vi "UI.vi"() -> ()   [LabVIEW 2015]
uses:
  Facade/cPAS Facade.lvclass
  Facade/Data.ctl
  Reusable/Commands/Command.lvclass
  Devices/Alicat/Session Based/Data/M/M data.lvclass
  Devices/Alicat/Session Based/Data/MC/MC Data.lvclass
  Reusable/GUI/Facade/GUI Facade.lvclass/GUI Facade.ctl
  Controls/Flags.ctl
  Reusable/Data/Read measTime.vi
  Reusable/GUI/Facade/GUI Facade.lvclass
  Reusable/Data/Data.lvclass
  Reusable/Error Logging/Error Logger.lvclass
panel:
  in  "swDispl":T1={"mDispl"=TRUE, "crdCtl"=FALSE, "pasCtl"=FALSE, "housekeeping"=FALSE, "crdRD"=FALSE, "pasSig"=FALSE, "power"=FALSE, "power 2"=FALSE, "power 3"=FALSE, "power 4"=FALSE}
  in  "saveRDs":bool
  out "Version":string
  in  "Sync Time":bool
  out "filter?":bool caption="Filter?"
  out "PAS Time Good":bool
  out "CRD Time Good":bool
  out "filtTime":timestamp caption="Last Filter Switch" format="%<%H:%M:%S>T"
  out "pasTime":timestamp caption="PAS Time" format="%<%H:%M:%S>T"
  out "crdTime":timestamp caption="CRD Time" format="%<%H:%M:%S>T"
  in  "filter":bool
  out "General Error":bool
  out "CRD Error":bool
  out "PAS Error":bool
  out "Saving":bool
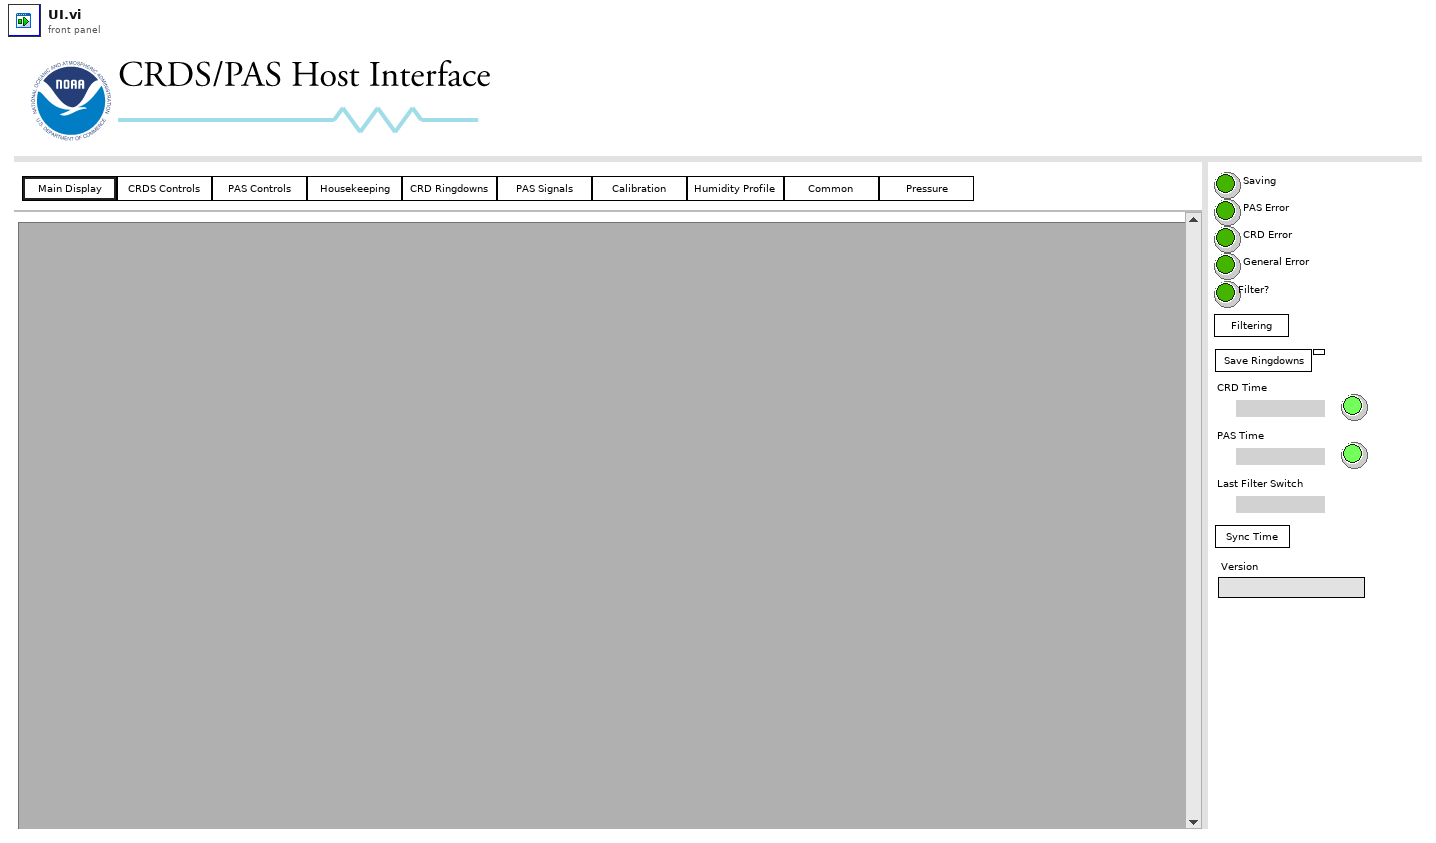
[diagram p1: front panel]
types:
  T1 = cluster{"mDispl":bool, "crdCtl":bool, "pasCtl":bool, "housekeeping":bool, "crdRD":bool, "pasSig":bool, "power":bool, "power 2":bool, "power 3":bool, "power 4":bool}
  T2 = enum8{"Enabled", "Disabled", "Disabled and Grayed Out"}
  T3 = typedef "cPAS Facade.lvclass/Data.ctl" = enum16{"PAS", "CRD", "CLAP"}
  T4 = typedef "Flags.ctl" = enum8{"Autospeaker", "Link cycles", "Autofilter", "O3 Cal", "Filter Position"}
  T5 = cluster{"[0]":bool, "[1]":bool, "[2]":bool, "[3]":bool, "[4]":bool, "[5]":bool, "[6]":bool, "[7]":bool, "[8]":bool, "[9]":bool}
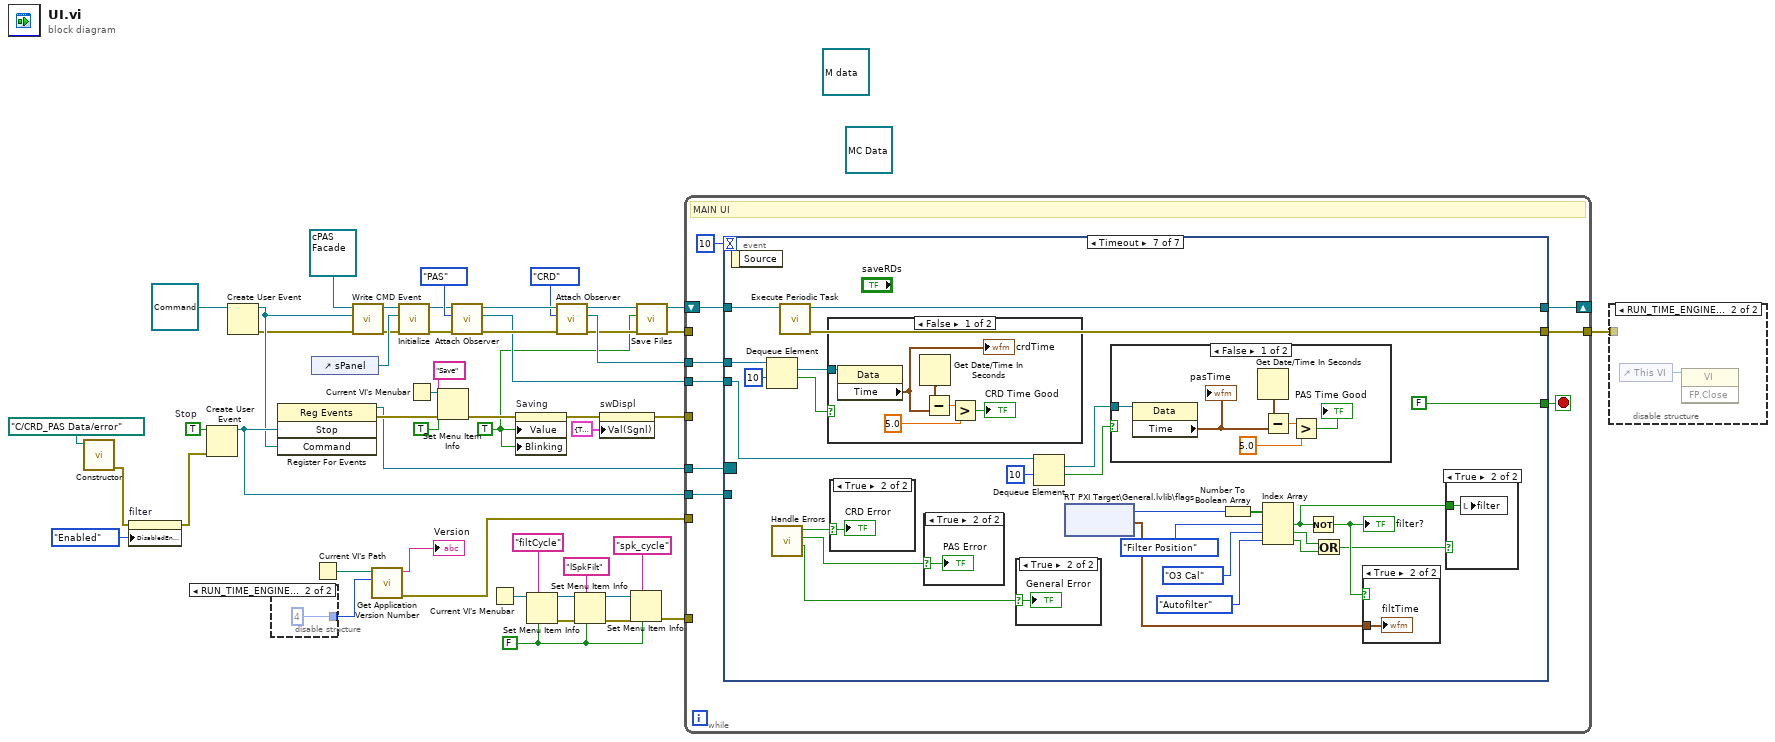
[diagram p0: block diagram]
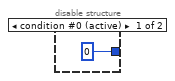
[diagram p2: hidden frame]
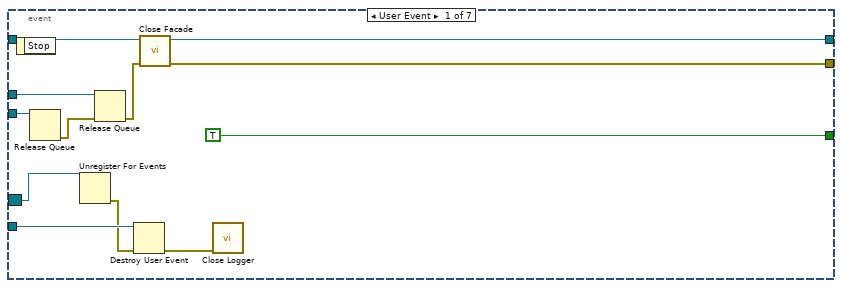
[diagram p4: hidden frame]
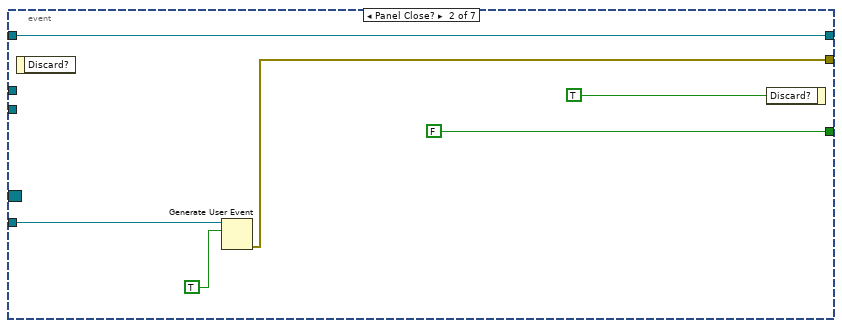
[diagram p5: hidden frame]
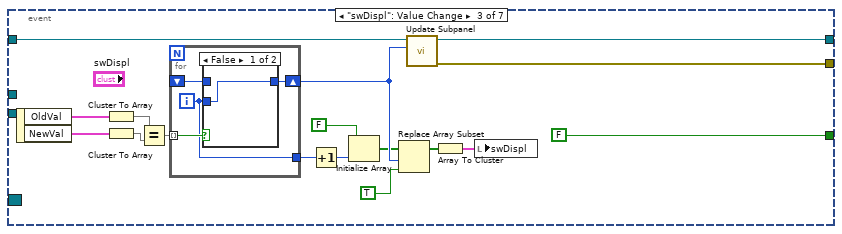
[diagram p6: hidden frame]
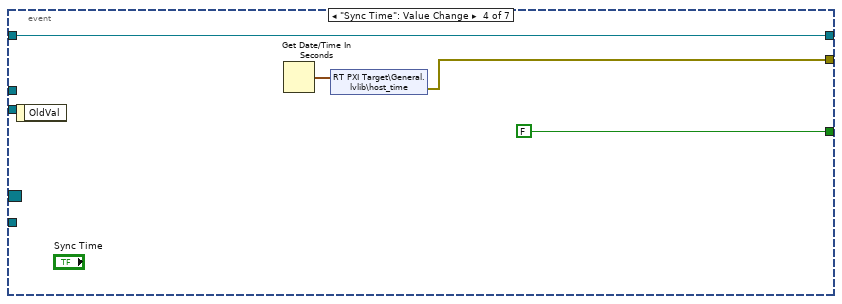
[diagram p8: hidden frame]
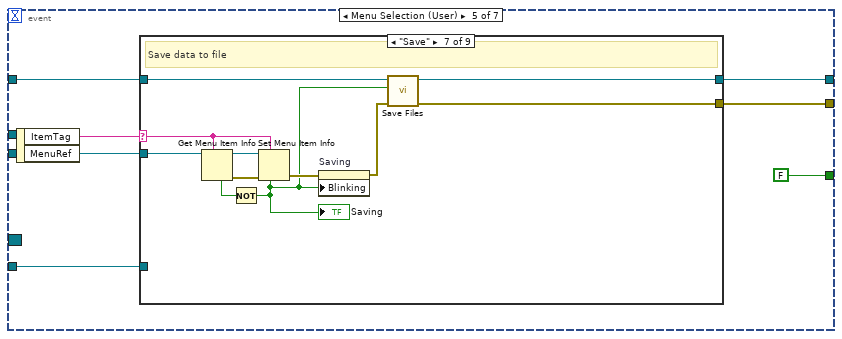
[diagram p9: hidden frame]
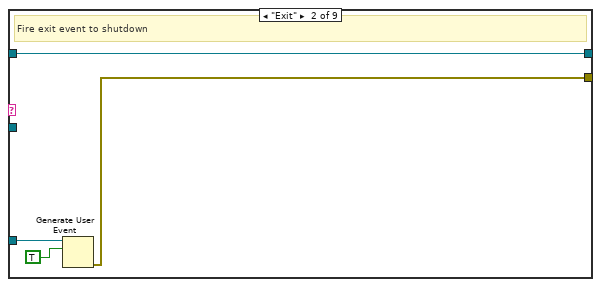
[diagram p11: hidden frame]
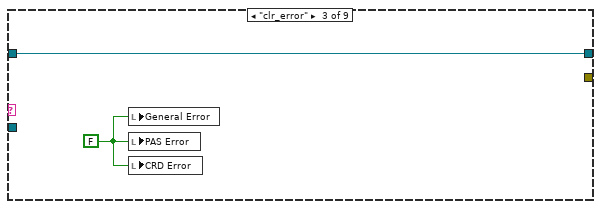
[diagram p12: hidden frame]
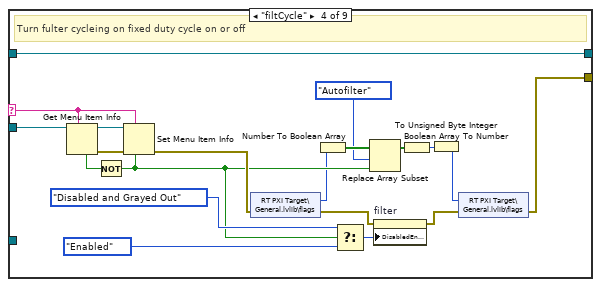
[diagram p13: hidden frame]
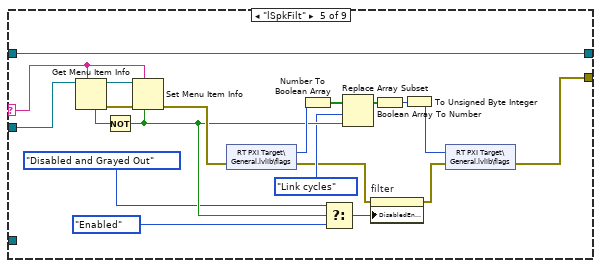
[diagram p14: hidden frame]
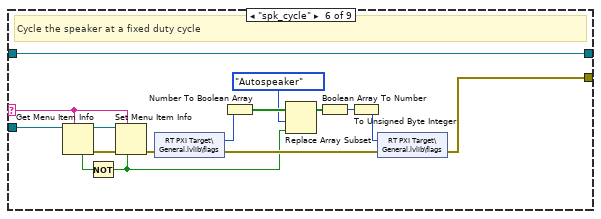
[diagram p15: hidden frame]
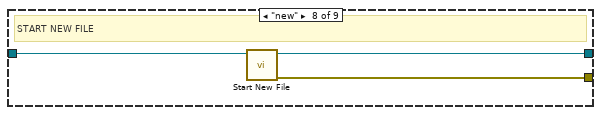
[diagram p16: hidden frame]
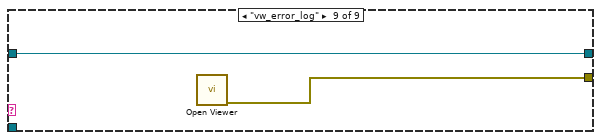
[diagram p17: hidden frame]
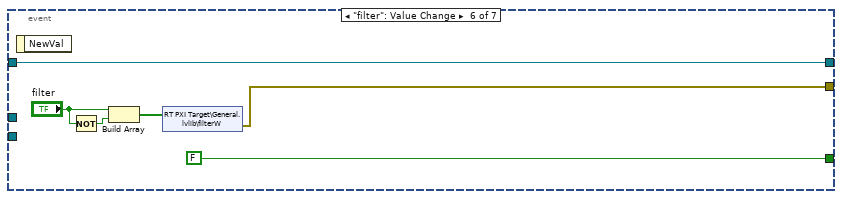
[diagram p18: hidden frame]
diagram:
  (unwired) refnum<class "MC Data.lvclass"> refnum ("MC Data")
  (unwired) refnum<class "M data.lvclass"> refnum ("M Data")
  w8 = FALSE ("checked")
  w39 = TRUE  # Stop
  w32 = TRUE ("Saving")
  n1 = call "Constructor.vi"("Main Path"=path "C:/CRD_PAS Data/error" ("Data Path")) -> ("error out"=w6:errorcluster)  [unwired: 10 in]
  n2 = property on="filter" class="Bool (strict)"(error in=w6, "DisabledEnum"=T2."Enabled" ("Disabled")) -> (error out=w17:errorcluster)  [unwired: 1 in, 1 out]
  n3 = Create User Event(user event datatype=w39, error in=w17) -> (user event=w37:refnum<user-event>)  [unwired: 1 out]
  n4 = Create User Event(user event datatype=refnum<class "Command.lvclass"> refnum ("Command")) -> (user event=w21:refnum<user-event>, error out=w19:errorcluster)  [unwired: 1 in]
  n5 = disable-structure shown="RUN_TIME_ENGINE==True" {
    disable-tunnel: [0 ("Number to Strip") 4 ("Number to Strip")] -> w4
    frame condition #0 (active) {
    }
    frame condition #1 {
    }
  }
  n6 = register-events(w37, w21) -> (reference out=w27:refnum<event-registration>, error out=w38:errorcluster)  [unwired: 2 in]
  n7 = control-ref of="sPanel"() -> (w46:refnum<vi>)
  n8 = Current VI's Path() -> (path=w5:path)
  n9 = call "Write CMD Event.vi"("error in (no error)"=w19, "CMD Event"=w21, "GUI Facade in"=refnum<class "cPAS Facade.lvclass"> refnum ("cPAS Facade")) -> ("error out"=w22:errorcluster, "GUI Facade out"=w23:refnum<class "cPAS Facade.lvclass">)  [unwired: 7 in]
  n10 = call "Get Application Version Number.vi"("Number to Strip"=w4, "Initial Path"=w5) -> ("error out"=w3:errorcluster, "Version"=→"Version":string)  [unwired: 8 in]
  n11 = call-dynamic "Initialize.vi"("error in"=w22, "sPanel"=w46, "GUI Facade in"=w23) -> ("error out"=w1:errorcluster, "GUI Facade out"=w20:refnum<class "cPAS Facade.lvclass">)  [unwired: 7 in]
  n12 = Current VI's Menubar() -> (w50:refnum<k9>)
  n13 = Set Menu Item Info(6:TRUE ("checked"), 7:"Save" ("item tag"), 8:w38, 11:w50) -> (0:w47:errorcluster)  [unwired: 3 in, 1 out]
  n14 = call "Attach Observer.vi"("error in"=w1, "Subject"=Data."PAS" ("Data"), "GUI Facade in"=w20) -> ("error out"=w44:errorcluster, "Observer"=w40:refnum<queue>, "GUI Facade out"=w45:refnum<class "cPAS Facade.lvclass">)  [unwired: 6 in]
  n15 = Current VI's Menubar() -> (w16:refnum<k9>)
  n16 = property on="Saving" class="Bool (strict)"(error in=w47, "Value"=w32, "Blinking"=w32) -> (error out=w30:errorcluster)  [unwired: 1 in, 1 out]
  n17 = Set Menu Item Info(6:w8, 7:"filtCycle" ("item tag"), 11:w16) -> (0:w12:errorcluster, 3:w13:refnum<k9>)  [unwired: 4 in]
  n18 = call "Attach Observer.vi"("error in"=w44, "Subject"=Data."CRD" ("Data"), "GUI Facade in"=w45) -> ("error out"=w34:errorcluster, "Observer"=w41:refnum<queue>, "GUI Facade out"=w36:refnum<class "cPAS Facade.lvclass">)  [unwired: 6 in]
  n19 = Set Menu Item Info(6:w8, 7:"lSpkFilt" ("item tag"), 8:w12, 11:w13) -> (0:w10:errorcluster, 3:w11:refnum<k9>)  [unwired: 3 in]
  n20 = property on="swDispl" class="Clust (strict)"(error in=w30, "Val(Sgnl)"=T1 {"mDispl"=TRUE, "crdCtl"=FALSE, "pasCtl"=FALSE, "housekeeping"=FALSE, "crdRD"=FALSE, "pasSig"=FALSE, "power"=FALSE, "power 2"=FALSE, "power 3"=FALSE, "power 4"=FALSE} ("Value (Signaling)")) -> (error out=w29:errorcluster)  [unwired: 1 in, 1 out]
  n21 = Set Menu Item Info(6:w8, 7:"spk_cycle" ("item tag"), 8:w10, 11:w11) -> (0:w7:errorcluster)  [unwired: 3 in, 1 out]
  n22 = call "Save Files.vi"("error in"=w34, "Write"=w32, "GUI Facade in"=w36) -> ("error out"=w33:errorcluster, "GUI Facade out"=w35:refnum<class "cPAS Facade.lvclass">)  [unwired: 7 in]
  n23 = while {
    shift-right: [w58] -> _
    shift-left: w35 -> [w59]
    tunnel: w41 -> [w57]
    tunnel: w40 -> [w56]
    tunnel: w27 -> [w55]
    tunnel: w37 -> [w54]
    tunnel: [w53] -> w28
    tunnel: w33 -> [_]
    tunnel: w29 -> [_]
    tunnel: w7 -> [_]
    tunnel: w3 -> [_]
    stop <- w61 stop-if-true
    # "MAIN UI"
    n24 = event shown="[6] Timeout" {
      selector: w55 -> [w65 _ _ _ _ _ _]
      dyn-events: _ -> [_ _ _ _ _ _ _]
      timeout: 10 -> [_ _ _ _ _ _ _]
      tunnel: [TRUE ("stop") FALSE ("stop") FALSE ("stop") FALSE ("stop") FALSE ("stop") FALSE ("stop") FALSE ("stop")] -> w61
      tunnel: [w71 w76 w92 w103 w111 w197 w223] -> w53
      tunnel: w59 -> [w72 w75 w93 w106 w110 w196 w224]
      tunnel: [w70 w75 w91 w106 w109 w196 w222] -> w58
      tunnel: w57 -> [w68 _ _ _ _ _ w218]
      tunnel: w56 -> [w69 _ _ _ _ _ w216]
      tunnel: w54 -> [w64 w77 _ _ w108 _ _]
      event User Event {
        n25 = event-data() -> ()  [unwired: 1 in, 1 out]
        n26 = Release Queue(queue=w69) -> (error out=w67:errorcluster)  [unwired: 2 in, 2 out]
        n27 = Unregister For Events(event registration refnum=w65) -> (error out=w63:errorcluster)  [unwired: 1 in]
        n28 = Release Queue(queue=w68, error in (no error)=w67) -> (error out=w66:errorcluster)  [unwired: 1 in, 2 out]
        n29 = Destroy User Event(user event=w64, error in=w63) -> (error out=w62:errorcluster)
        n30 = call-dynamic "Close Facade.vi"("error in"=w66, "cPAS Facade in"=w72) -> ("error out"=w71:errorcluster, "cPAS Facade out"=w70:refnum<class "cPAS Facade.lvclass">)  [unwired: 8 in]
        n31 = call "Close Logger.vi"("error in"=w62) -> ()  [unwired: 9 in, 2 out]
      }
      event Panel Close? {
        n32 = event-data() -> ()  [unwired: 1 in, 1 out]
        n33 = Generate User Event(user event=w77, event data cluster=TRUE ("event data")) -> (error out=w76:errorcluster)  [unwired: 2 in, 1 out]
        n34 = event-data("Discard?"=TRUE) -> ()  [unwired: 1 in, 1 out]
      }
      event "swDispl": Value Change {
        n35 = event-data() -> ("OldVal"=w96:T1, "NewVal"=w95:T1)  [unwired: 1 in]
        n36 = Cluster To Array(cluster=w96) -> (array=w89:bool[])
        n37 = Cluster To Array(cluster=w95) -> (array=w90:bool[])
        n38 = Equal?(x=w89, y=w90) -> (x = y?=w94:bool[])
        n39 = for {
          tunnel: w94 -> [w100] mode=indexing
          shift-right: [w99] -> w85
          shift-left: _ -> [w98]
          tunnel: [w97] -> w88
          i -> [w97]
          n40 = case shown="False" w100 {
            tunnel: w97 -> [w101 _]
            tunnel: [w101 w102] -> w99
            tunnel: w98 -> [_ w102]
            frame False {
            }
            frame True {
            }
          }
        }
        n41 = Increment(x=w88) -> (x+1=w87:i32)
        n42 = Initialize Array(FALSE, w87) -> (w84:bool[])
        n43 = Replace Array Subset(array=w84, new element=TRUE ("new element/subarray"), index=w85) -> (w82:bool[])
        n44 = call "Update Subpanel.vi"("sPanel"=w85, "GUI Facade in"=w93) -> ("error out"=w92:errorcluster, "GUI Facade out"=w91:refnum<class "cPAS Facade.lvclass">)  [unwired: 8 in]
        n45 = Array To Cluster(array=w82) -> (cluster=w81:T5)
        n46 = local write "swDispl"(w81) -> ()
      }
      event "Sync Time": Value Change {
        n47 = event-data() -> ()  [unwired: 1 in, 1 out]
        n48 = Get Date/Time In Seconds() -> (seconds since 1Jan1904=w104:timestamp)
        n49 = shared-variable "RT PXI Target\\General.lvlib\\host_time"(w104) -> (error out=w103:errorcluster)  [unwired: 1 in]
      }
      event Menu Selection (User) {
        n50 = event-data() -> ("ItemTag"=w112:string, "MenuRef"=w113:refnum<k9>)  [unwired: 1 in]
        n51 = case shown="\"Save\"" w112 {
          selector: w112 -> [_ _ _ w136 w147 w165 w182 _ _]
          tunnel: w113 -> [_ _ _ w135 w146 w166 w183 _ _]
          tunnel: [_ w115 _ w133 w144 w164 w177 w188 w191] -> w111
          tunnel: [w114 w118 w119 w140 w145 w163 w180 w189 w192] -> w109
          tunnel: w110 -> [w114 w118 w119 w140 w145 w163 w181 w190 w192]
          tunnel: w108 -> [_ w117 _ _ _ _ _ _ _]
          frame "NULL", Default {
            # "Do Nothing"
          }
          frame "Exit" {
            # "Fire exit event to shutdown"
            n52 = Generate User Event(user event=w117, event data cluster=TRUE ("event data")) -> (error out=w115:errorcluster)  [unwired: 2 in, 1 out]
          }
          frame "clr_error" {
            w120 = FALSE
            n53 = local write "General Error"(w120) -> ()
            n54 = local write "PAS Error"(w120) -> ()
            n55 = local write "CRD Error"(w120) -> ()
          }
          frame "filtCycle" {
            # "Turn fulter cycleing on fixed duty cycle on or off"
            n56 = Get Menu Item Info(7:w136, 11:w135) -> (0:w137:errorcluster, 3:w138:refnum<k9>, 4:w139:bool)  [unwired: 1 in, 4 out]
            n57 = Not(x=w139) -> (.not. x?=w129:bool)
            n58 = Set Menu Item Info(6:w129, 7:w136, 8:w137, 11:w138) -> (0:w134:errorcluster)  [unwired: 3 in, 1 out]
            n59 = shared-variable "RT PXI Target\\General.lvlib\\flags"(error in=w134) -> (w124:u8, error out=w122:errorcluster)
            n60 = Number To Boolean Array(number=w124) -> (Boolean array=w125:bool[])
            n61 = Select(t=T2."Disabled and Grayed Out", s=w129, f=T2."Enabled" ("Disabled")) -> (s? t:f=w130:T2)
            n62 = Replace Array Subset(array=w125, new element=w129, index=Flags."Autofilter" ("Flags")) -> (w126:bool[])
            n63 = property on="filter" class="Bool (strict)"(error in=w122, "DisabledEnum"=w130) -> (error out=w121:errorcluster)  [unwired: 1 in, 1 out]
            n64 = Boolean Array To Number(Boolean array=w126) -> (number=w127:u32)
            n65 = To Unsigned Byte Integer(number=w127) -> (unsigned 8bit integer=w128:u8)
            n66 = shared-variable "RT PXI Target\\General.lvlib\\flags"(w128, error in=w121) -> (error out=w133:errorcluster)
          }
          frame "lSpkFilt" {
            n67 = Get Menu Item Info(7:w147, 11:w146) -> (0:w158:errorcluster, 3:w159:refnum<k9>, 4:w160:bool)  [unwired: 1 in, 4 out]
            n68 = Not(x=w160) -> (.not. x?=w150:bool)
            n69 = Set Menu Item Info(6:w150, 7:w147, 8:w158, 11:w159) -> (0:w152:errorcluster)  [unwired: 3 in, 1 out]
            n70 = shared-variable "RT PXI Target\\General.lvlib\\flags"(error in=w152) -> (w153:u8, error out=w142:errorcluster)
            n71 = Number To Boolean Array(number=w153) -> (Boolean array=w154:bool[])
            n72 = Select(t=T2."Disabled and Grayed Out", s=w150, f=T2."Enabled" ("Disabled")) -> (s? t:f=w148:T2)
            n73 = Replace Array Subset(array=w154, new element=w150, index=Flags."Link cycles" ("Flags")) -> (w155:bool[])
            n74 = property on="filter" class="Bool (strict)"(error in=w142, "DisabledEnum"=w148) -> (error out=w141:errorcluster)  [unwired: 1 in, 1 out]
            n75 = Boolean Array To Number(Boolean array=w155) -> (number=w156:u32)
            n76 = To Unsigned Byte Integer(number=w156) -> (unsigned 8bit integer=w157:u8)
            n77 = shared-variable "RT PXI Target\\General.lvlib\\flags"(w157, error in=w141) -> (error out=w144:errorcluster)
          }
          frame "spk_cycle" {
            # "Cycle the speaker at a fixed duty cycle"
            n78 = Get Menu Item Info(7:w165, 11:w166) -> (0:w174:errorcluster, 3:w176:refnum<k9>, 4:w175:bool)  [unwired: 1 in, 4 out]
            n79 = Not(x=w175) -> (.not. x?=w162:bool)
            n80 = Set Menu Item Info(6:w162, 7:w165, 8:w174, 11:w176) -> (0:w167:errorcluster)  [unwired: 3 in, 1 out]
            n81 = shared-variable "RT PXI Target\\General.lvlib\\flags"(error in=w167) -> (w172:u8, error out=w173:errorcluster)
            n82 = Number To Boolean Array(number=w172) -> (Boolean array=w171:bool[])
            n83 = Replace Array Subset(array=w171, new element=w162, index=Flags."Autospeaker" ("Flags")) -> (w170:bool[])
            n84 = Boolean Array To Number(Boolean array=w170) -> (number=w169:u32)
            n85 = To Unsigned Byte Integer(number=w169) -> (unsigned 8bit integer=w168:u8)
            n86 = shared-variable "RT PXI Target\\General.lvlib\\flags"(w168, error in=w173) -> (error out=w164:errorcluster)
          }
          frame "Save" {
            # "Save data to file"
            n87 = Get Menu Item Info(7:w182, 11:w183) -> (0:w185:errorcluster, 3:w186:refnum<k9>, 4:w187:bool)  [unwired: 1 in, 4 out]
            n88 = Not(x=w187) -> (.not. x?=w179:bool)
            "Saving" <- w179
            n89 = Set Menu Item Info(6:w179, 7:w182, 8:w185, 11:w186) -> (0:w184:errorcluster)  [unwired: 3 in, 1 out]
            n90 = property on="Saving" class="Bool (strict)"(error in=w184, "Blinking"=w179) -> (error out=w178:errorcluster)  [unwired: 1 in, 1 out]
            n91 = call "Save Files.vi"("error in"=w178, "Write"=w179, "GUI Facade in"=w181) -> ("error out"=w177:errorcluster, "GUI Facade out"=w180:refnum<class "cPAS Facade.lvclass">)  [unwired: 7 in]
          }
          frame "new" {
            # "START NEW FILE"
            n92 = call "Start New File.vi"("GUI Facade in"=w190) -> ("error out"=w188:errorcluster, "GUI Facade out"=w189:refnum<class "cPAS Facade.lvclass">)  [unwired: 9 in]
          }
          frame "vw_error_log" {
            n93 = call "Open Viewer.vi"() -> ("error out"=w191:errorcluster)  [unwired: 11 in]
          }
        }
      }
      event "filter": Value Change {
        n94 = event-data() -> ()  [unwired: 1 in, 1 out]
        n95 = Not(x="filter") -> (.not. x?=w194:bool)
        n96 = Build Array("filter", w194) -> (w198:bool[])
        n97 = shared-variable "RT PXI Target\\General.lvlib\\filterW"(w198) -> (error out=w197:errorcluster)  [unwired: 1 in]
      }
      event Timeout {
        n98 = event-data() -> ()  [unwired: 1 in, 1 out]
        n99 = Dequeue Element(queue=w218, timeout in ms (-1)=10) -> (element=w217:refnum<data-value>, timed out?=w211:bool)  [unwired: 1 in, 2 out]
        n100 = call "Handle Errors.vi"() -> ("General"=w208:bool, "PAS"=w207:bool, "CRD"=w206:bool)  [unwired: 9 in]
        n101 = call-dynamic "Execute Periodic Task.vi"("GUI Facade in"=w224) -> ("error out"=w223:errorcluster, "GUI Facade out"=w222:refnum<class "cPAS Facade.lvclass">)  [unwired: 9 in]
        n102 = case shown="False" w211 {
          tunnel: w217 -> [w231 _]
          frame False {
            n103 = property class="Data"(reference=w231) -> ("Time"=w227:timestamp)  [unwired: 1 in, 2 out]
            "crdTime" <- w227
            n104 = Get Date/Time In Seconds() -> (seconds since 1Jan1904=w228:timestamp)
            n105 = Subtract(x=w228, y=w227) -> (x-y=w229:dbl)
            n106 = Greater?(x=w229, y=5.0) -> (0:→"CRD Time Good":bool)
          }
          frame True {
          }
        }
        n107 = case shown="True" w206 {
          selector: w206 -> [_ w238]
          frame False {
          }
          frame True {
            "CRD Error" <- w238
          }
        }
        n108 = case shown="True" w207 {
          selector: w207 -> [_ w240]
          frame False {
          }
          frame True {
            "PAS Error" <- w240
          }
        }
        n109 = case shown="True" w208 {
          selector: w208 -> [_ w239]
          frame False {
          }
          frame True {
            "General Error" <- w239
          }
        }
        n110 = Dequeue Element(queue=w216, timeout in ms (-1)=10) -> (element=w215:refnum<data-value>, timed out?=w212:bool)  [unwired: 1 in, 2 out]
        n111 = shared-variable "RT PXI Target\\General.lvlib\\flags"() -> (w221:u8, w219:timestamp)  [unwired: 1 in, 1 out]
        n112 = case shown="False" w212 {
          tunnel: w215 -> [w237 _]
          frame False {
            n113 = property class="Data"(reference=w237) -> ("Time"=w235:timestamp)  [unwired: 1 in, 2 out]
            "pasTime" <- w235
            n114 = Get Date/Time In Seconds() -> (seconds since 1Jan1904=w234:timestamp)
            n115 = Subtract(x=w234, y=w235) -> (x-y=w233:dbl)
            n116 = Greater?(x=w233, y=5.0) -> (0:→"PAS Time Good":bool)
          }
          frame True {
          }
        }
        n117 = Number To Boolean Array(number=w221) -> (Boolean array=w220:bool[])
        n118 = Index Array(array=w220, index #1=Flags."Filter Position" ("Flags"), index #2=Flags."O3 Cal" ("Flags"), index #3=Flags."Autofilter" ("Flags")) -> (element #1=w209:bool, element #2=w201:bool, element #3=w200:bool)
        n119 = Not(x=w209) -> (.not. x?=w205:bool)
        "filter?" <- w205
        n120 = Or(x=w201, y=w200) -> (x .or. y?=w199:bool)
        n121 = case shown="True" w205 {
          tunnel: w219 -> [_ w241]
          frame False {
          }
          frame True {
            "filtTime" <- w241
          }
        }
        n122 = case shown="True" w199 {
          tunnel: w209 -> [_ w225]
          frame False {
          }
          frame True {
            n123 = local write "filter"(w225) -> ()
          }
        }
      }
    }
  }
  n124 = disable-structure shown="RUN_TIME_ENGINE==True" {
    disable-tunnel: w28 -> [_ _]
    frame condition #0 (active) {
    }
    frame condition #1 {
      n125 = control-ref of="This VI"() -> (w242:refnum<vi>)
      n126 = invoke class="VI" method="FP.Close"(reference=w242) -> ()  [unwired: 2 in, 3 out]
    }
  }
